vi "Write ConvBox Handler.vi"(8 "error in (no error)":errorcluster, 9 "Data Length":string, 10 "Data":string, 11 "Listener in":refnum<class "Listener.lvclass">) -> (0 "error out":errorcluster, 3 "Listener out":refnum<class "Listener.lvclass">)   [LabVIEW 2019, in "Listener.lvclass"]
uses:
  Listener.lvclass
  Listener.lvclass/Listener.ctl
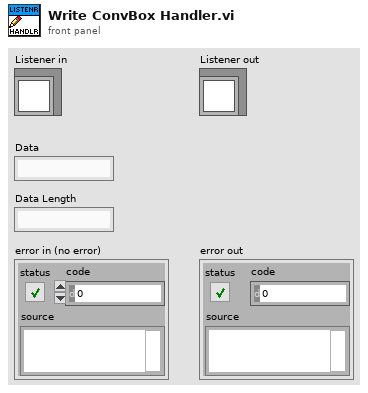
[diagram p1: front panel]
types:
  T1 = typedef "Listener.lvclass/RS-xxx To GPIB ConvBox Data Structure.ctl" = cluster{"Data":string, "Command Messages Read":string[], "Address":string, "Data Length":u32}
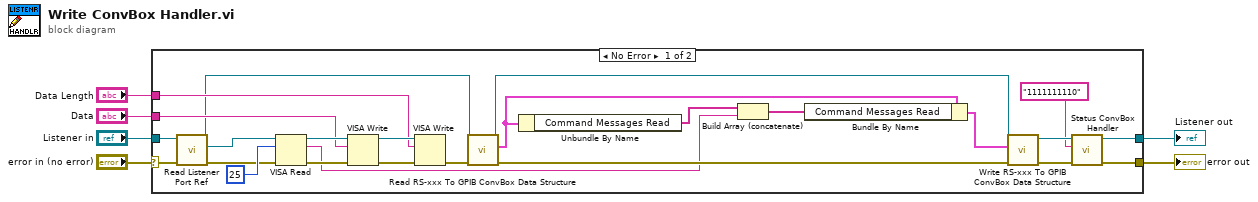
[diagram p0: block diagram]
diagram:
  n1 = case shown="No Error" "error in (no error)" {
    selector: "error in (no error)" -> [w22 w33]
    tunnel: [w27 w33] -> w6
    tunnel: "Data" -> [w26 _]
    tunnel: "Data Length" -> [w23 _]
    tunnel: "Listener in" -> [w21 w32]
    tunnel: [w28 w32] -> w1
    frame No Error {
      n2 = call "Read Listener Port Ref.vi"("error in (no error)"=w22, "Listener in"=w21) -> ("error out"=w20:errorcluster, "Listener Port Ref"=w19:refnum<visa-resource-name>, "Listener out"=w17:refnum<class "Listener.lvclass">)  [unwired: 7 in]
      n3 = VISA Read(VISA resource name=w19, byte count=u32 25, error in (no error)=w20) -> (VISA resource name out=w31:refnum<visa-resource-name>, read buffer=w8:string, error out=w30:errorcluster)  [unwired: 1 out]
      n4 = VISA Write(VISA resource name=w31, write buffer=w26, error in (no error)=w30) -> (VISA resource name out=w25:refnum<visa-resource-name>, error out=w24:errorcluster)  [unwired: 1 out]
      n5 = VISA Write(VISA resource name=w25, write buffer=w23, error in (no error)=w24) -> (error out=w18:errorcluster)  [unwired: 2 out]
      n6 = call-dynamic "Read RS-xxx To GPIB ConvBox Data Structure.vi"("error in (no error)"=w18, "Listener in"=w17) -> ("error out"=w16:errorcluster, "RS-xxx To GPIB ConvBox Data Structure"=w13:T1, "Listener out"=w15:refnum<class "Listener.lvclass">)  [unwired: 7 in]
      n7 = Unbundle By Name(w13) -> ("Command Messages Read"=w9:string[])
      n8 = Build Array (concatenate)(w9, w8) -> (w7:string[])
      n9 = Bundle By Name(cluster=w13, "Command Messages Read"=w7) -> (w12:T1)
      n10 = call-dynamic "Write RS-xxx To GPIB ConvBox Data Structure.vi"("error in (no error)"=w16, "RS-xxx To GPIB ConvBox Data Structure"=w12, "Listener in"=w15) -> ("error out"=w14:errorcluster, "Listener out"=w11:refnum<class "Listener.lvclass">)  [unwired: 7 in]
      n11 = call "Status ConvBox Handler.vi"("error in(no error)"=w14, "Value In"="1111111110" ("write buffer"), "Listener in"=w11) -> ("error out"=w27:errorcluster, "Listener out"=w28:refnum<class "Listener.lvclass">)  [unwired: 7 in]
    }
    frame Error {
    }
  }
  "error out" <- w6
  "Listener out" <- w1
